vi "TestHB_Emb_3.vi"() -> ()   [LabVIEW 2012]
doc: "SciScan 1.2 160622"
uses:
  Custom Controls and Typedefs/Heartbeat information cluster.ctl
  Custom Controls and Typedefs/Heartbeat Event Source.ctl
  Custom Controls/Heartbeat_States.ctl
  Custom Controls and Typedefs/HB_Error Conditions Cluster.ctl
  SubVIs/Master Slave messaging Flags.ctl
  SubVIs/Heartbeat state manager Input VI names.ctl
  Custom Controls and Typedefs/HB Actionable Event.ctl
  Custom Controls and Typedefs/HFG Commands.ctl
panel:
  out "Slave Completions Received":i32
  out "Master Instructions Issued":i32
  out "Received String":string
  out "No of Strings received":i32
  in  "stop":bool
  out "Master-Slave messaging Flags":T1={"Instruction available"=TRUE, "Slave action completed"=TRUE, "Slave Ready?"=FALSE}
  out "Error conditions Cluster":T2
  out "Heartbeat information cluster":T3
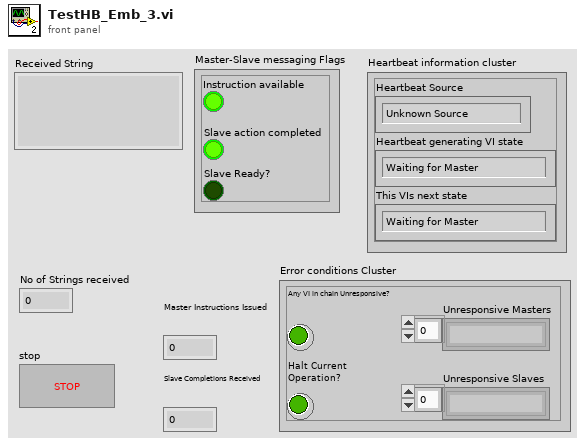
[diagram p1: front panel]
types:
  T1 = typedef "Master Slave messaging Flags.ctl" = cluster{"Instruction available":bool, "Slave action completed":bool, "Slave Ready?":bool}
  T2 = typedef "HB_Error Conditions Cluster.ctl" = cluster{"Any VI in chain Unresponsive?":bool, "Halt Current Operation?":bool, "Unresponsive Masters":string[], "Unresponsive Slaves":string[]}
  T3 = typedef "Heartbeat information cluster.ctl" = cluster{"Heartbeat Source":T4, "Heartbeat generating VI state":T5, "This VIs next state":T5}
  T4 = typedef "Heartbeat Event Source.ctl" = enum16{"Unknown Source", "Timeout", "This VI", "Master", "Slave"}
  T5 = typedef "Heartbeat_States.ctl" = enum16{"Waiting for Master", "Instruction Issued", "Waiting for Slave Completion", "Completed", "Cancelled", "Failed", "Broken Link"}
  T6 = typedef "HB Actionable Event.ctl" = enum16{"Master instruction event", "Slave ready event", "Slave unavailable event", "Cancelled or Failed event", "Slave action complete event", "QUIT", "Broken Link", "Recovered from Broken Link"}
  T7 = typedef "Heartbeat state manager Input VI names.ctl" = cluster{"Current VI name":string, "Master VI Names":string[], "Slave VI Names":string[]}
  T8 = typedef "HFG Commands.ctl" = enum16{"Set", "Get", "Initialize"}
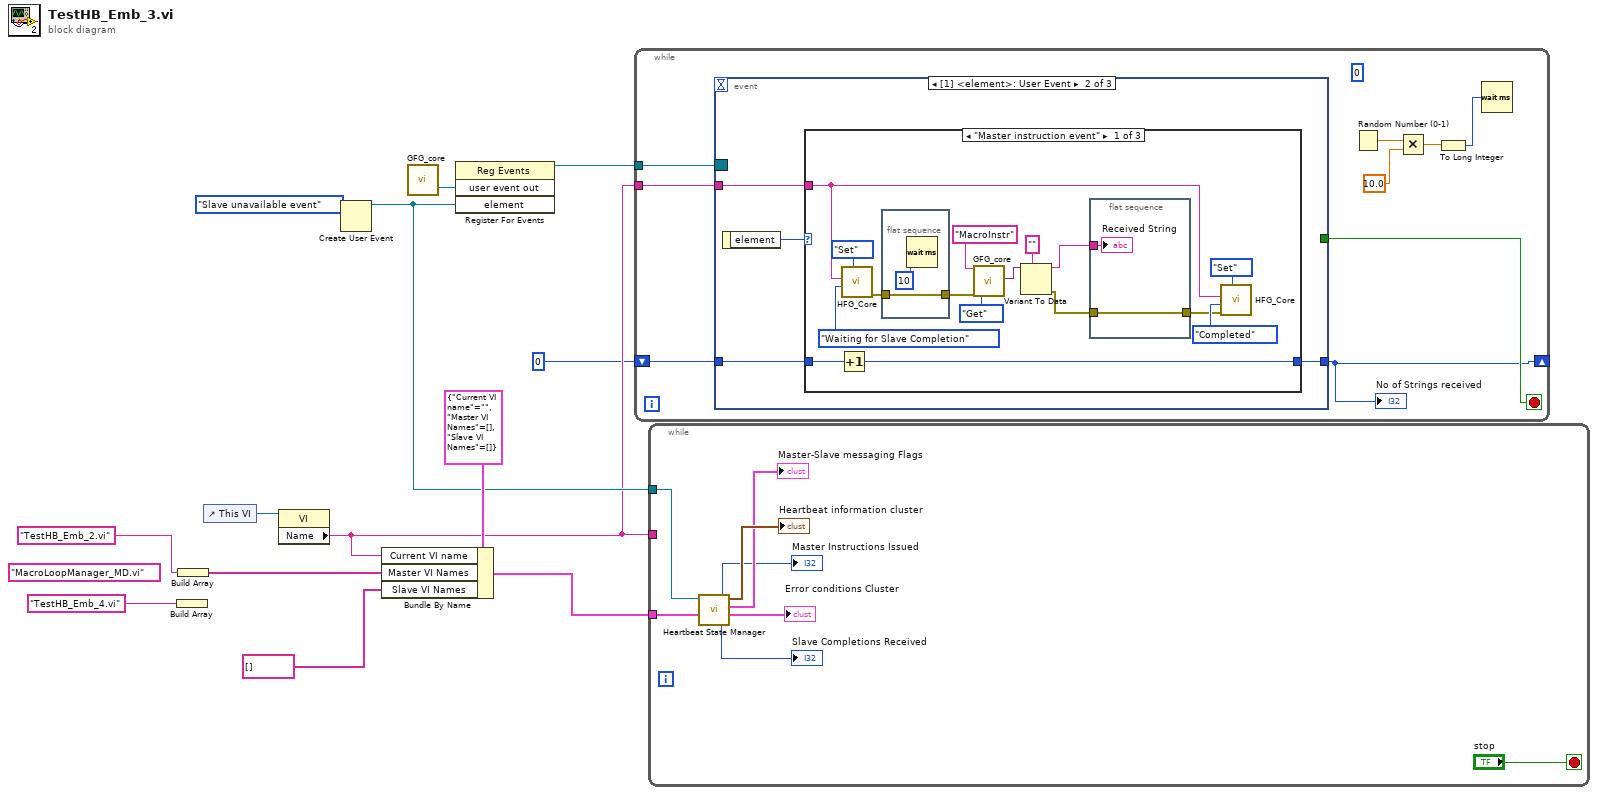
[diagram p0: block diagram]
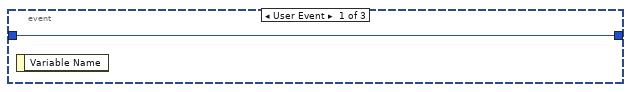
[diagram p2: hidden frame]
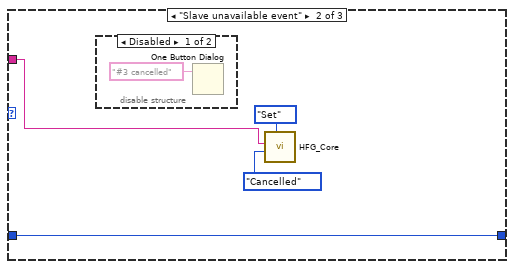
[diagram p3: hidden frame]
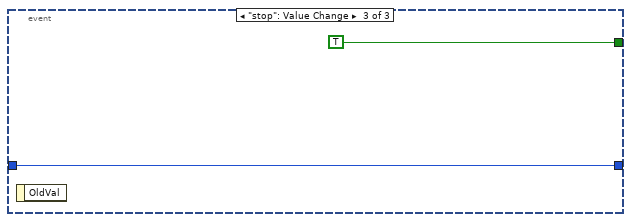
[diagram p6: hidden frame]
diagram:
  (unwired) "MacroLoopManager_MD.vi"
  n1 = Build Array("TestHB_Emb_4.vi") -> ()  [unwired: 1 out]
  n2 = Build Array("TestHB_Emb_2.vi") -> (w7:string[])
  n3 = control-ref of="This VI"() -> (w11:refnum<vi>)
  n4 = property class="VI"(reference=w11) -> ("Name"=w3:string)  [unwired: 1 in, 2 out]
  n5 = Create User Event(user event datatype=HB_Actionable_Event."Slave unavailable event" ("element")) -> (user event=w4:refnum<user-event>)  [unwired: 1 in, 1 out]
  n6 = Bundle By Name(cluster=T7 {"Current VI name"="", "Master VI Names"=[], "Slave VI Names"=[]} ("Heartbeat state manager Input VI names 2"), "Current VI name"=w3, "Master VI Names"=w7, "Slave VI Names"=string[] []) -> (w10:T7)
  n7 = call "GFG_core.vi"() -> ("user event out"=w9:refnum<user-event>)  [unwired: 13 in, 6 out]
  n8 = register-events(w9, w4) -> (reference out=w8:refnum<event-registration>)  [unwired: 2 in, 1 out]
  n9 = while {
    tunnel: w8 -> [w22]
    tunnel: w3 -> [w20]
    shift-right: [w18] -> _
    shift-left: 0 -> [w19]
    stop <- w21 stop-if-true
    (unwired) u32 0 ("milliseconds to wait")
    n10 = event shown="[1] <element>: User Event" {
      selector: w22 -> [_ _ _]
      dyn-events: _ -> [_ _ _]
      timeout: _ -> [_ _ _]
      tunnel: [_ _ TRUE] -> w21
      tunnel: w20 -> [_ w26 _]
      tunnel: w19 -> [w23 w25 w54]
      tunnel: [w23 w24 w54] -> w18
      event User Event {
        n11 = event-data() -> ()  [unwired: 1 in, 1 out]
      }
      event User Event {
        n12 = event-data() -> ("element"=w27:T6)  [unwired: 1 in]
        n13 = case shown="\"Master instruction event\"" w27 {
          tunnel: w26 -> [w30 w48 _]
          tunnel: w25 -> [w34 w51 w53]
          tunnel: [w33 w51 w53] -> w24
          frame "Master instruction event" {
            n14 = Increment(x=w34) -> (x+1=w33:i32)
            n15 = call "HFG_Core.vi"("HFG Commands"=HFG_Commands."Set", "Heartbeat state IN"=Heartbeat_States."Waiting for Slave Completion", "VI Name (Calling VIs name by default)"=w30) -> ("Error Out"=w29:errorcluster)  [unwired: 5 in, 3 out]
            n16 = flat-sequence {
              tunnel: w29 -> [w45]
              tunnel: [w45] -> w28
              frame #0 {
                n17 = Wait (ms)(milliseconds to wait=u32 10) -> ()  [unwired: 1 out]
              }
            }
            n18 = call "GFG_core.vi"("Variable Name in"="MacroInstr", "error in (no error)"=w28, "Action"=enum16{"Init", "Set", "Get", "Clear"}."Get") -> ("Variant Out"=w42:variant)  [unwired: 10 in, 6 out]
            n19 = Variant To Data(type="", Variant=w42) -> (data=w37:string, error out=w36:errorcluster)  [unwired: 1 in]
            n20 = flat-sequence {
              tunnel: w37 -> [w46]
              tunnel: w36 -> [w47]
              tunnel: [w47] -> w35
              frame #0 {
                "Received String" <- w46
              }
            }
            n21 = call "HFG_Core.vi"("HFG Commands"=HFG_Commands."Set", "Error In"=w35, "Heartbeat state IN"=Heartbeat_States."Completed", "VI Name (Calling VIs name by default)"=w30) -> ()  [unwired: 4 in, 4 out]
          }
          frame "Slave unavailable event" {
            n22 = disable-structure shown="Disabled" {
              frame Disabled {
                n23 = One Button Dialog(message="#3 cancelled") -> ()  [unwired: 1 in, 1 out]
              }
              frame Enabled {
              }
            }
            n24 = call "HFG_Core.vi"("HFG Commands"=HFG_Commands."Set", "Heartbeat state IN"=Heartbeat_States."Cancelled", "VI Name (Calling VIs name by default)"=w48) -> ()  [unwired: 5 in, 4 out]
          }
          frame Default {
          }
        }
      }
      event "stop": Value Change {
        n25 = event-data() -> ()  [unwired: 1 in, 1 out]
      }
    }
    "No of Strings received" <- w18
    n26 = Random Number (0-1)() -> (number: 0 to 1=w17:dbl)
    n27 = Multiply(x=w17, y=10.0) -> (x*y=w15:dbl)
    n28 = To Long Integer(number=w15) -> (32bit integer=w14:i32)
    n29 = Wait (ms)(milliseconds to wait=w14) -> ()  [unwired: 1 out]
  }
  n30 = while {
    tunnel: w10 -> [w63]
    tunnel: w4 -> [w58]
    tunnel: w3 -> [_]
    stop <- "stop" stop-if-true
    n31 = call "Heartbeat State Manager.vi"("Heartbeat state manager Input VI names"=w63, "HB Command Event IN"=w58) -> ("Error conditions Cluster"=→"Error conditions Cluster":T2, "Master-Slave messaging Flags"=→"Master-Slave messaging Flags":T1, "Heartbeat information cluster"=→"Heartbeat information cluster":T3, "Slave Completions Received"=→"Slave Completions Received":i32, "Master Instructions Issued"=→"Master Instructions Issued":i32)  [unwired: 4 in, 1 out]
  }
